vi "Verify Digraph for Simulation Mappings.vi"() -> (3 "test passed":bool)   [LabVIEW 2015]
uses:
  GraphViz Mapping Visualizer.lvlib
  <vilib>/NI/Tag Bus/tag/Data Type.ctl
  <vilib>/NI/Tag Bus/tag/tag descriptor.lvclass
panel:
  out "digraph output":string
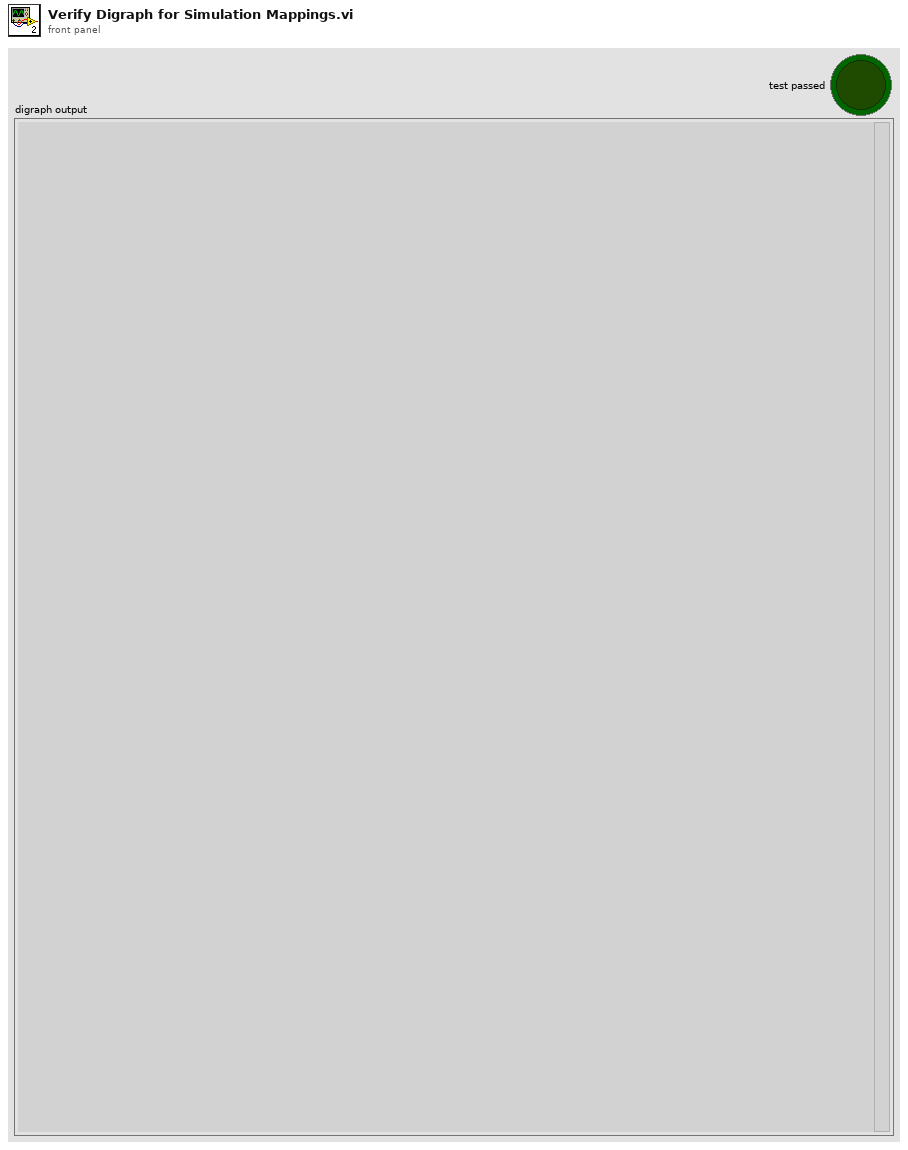
[diagram p1: front panel]
types:
  T1 = cluster{"Instance ID":string, "name":string, "default value string":string, "index":i32}[]
  T2 = typedef "tag bus.lvlib/tag descriptor.lvclass/Data Type.ctl" = enum16{"Double", "Single", "I64", "I32", "I16", "I8", "U64", "U32", "U16", "U8", "Boolean", "String", "Array of Double", "Array of Single", "Array of I64", "Array of I32", "Array of I16", "Array of I8", "Array of U64", "Array of U32", "Array of U16", "Array of U8", "Array of Boolean", "Array of String"}
  T3 = cluster{"name":string, "data type":T2, "writer":string, "readers":string[]}[]
  T4 = cluster{"display strings and indices":cluster{"Instance ID":string, "name":string, "default value string":string, "index":i32}[], "display strings and indices":cluster{"Instance ID":string, "name":string, "default value string":string, "index":i32}[]}
  T5 = typedef "GraphViz Mapping Visualizer.lvlib/Channel to Port Pair.ctl" = cluster{"Channel Name":string, "Node:Port":string}
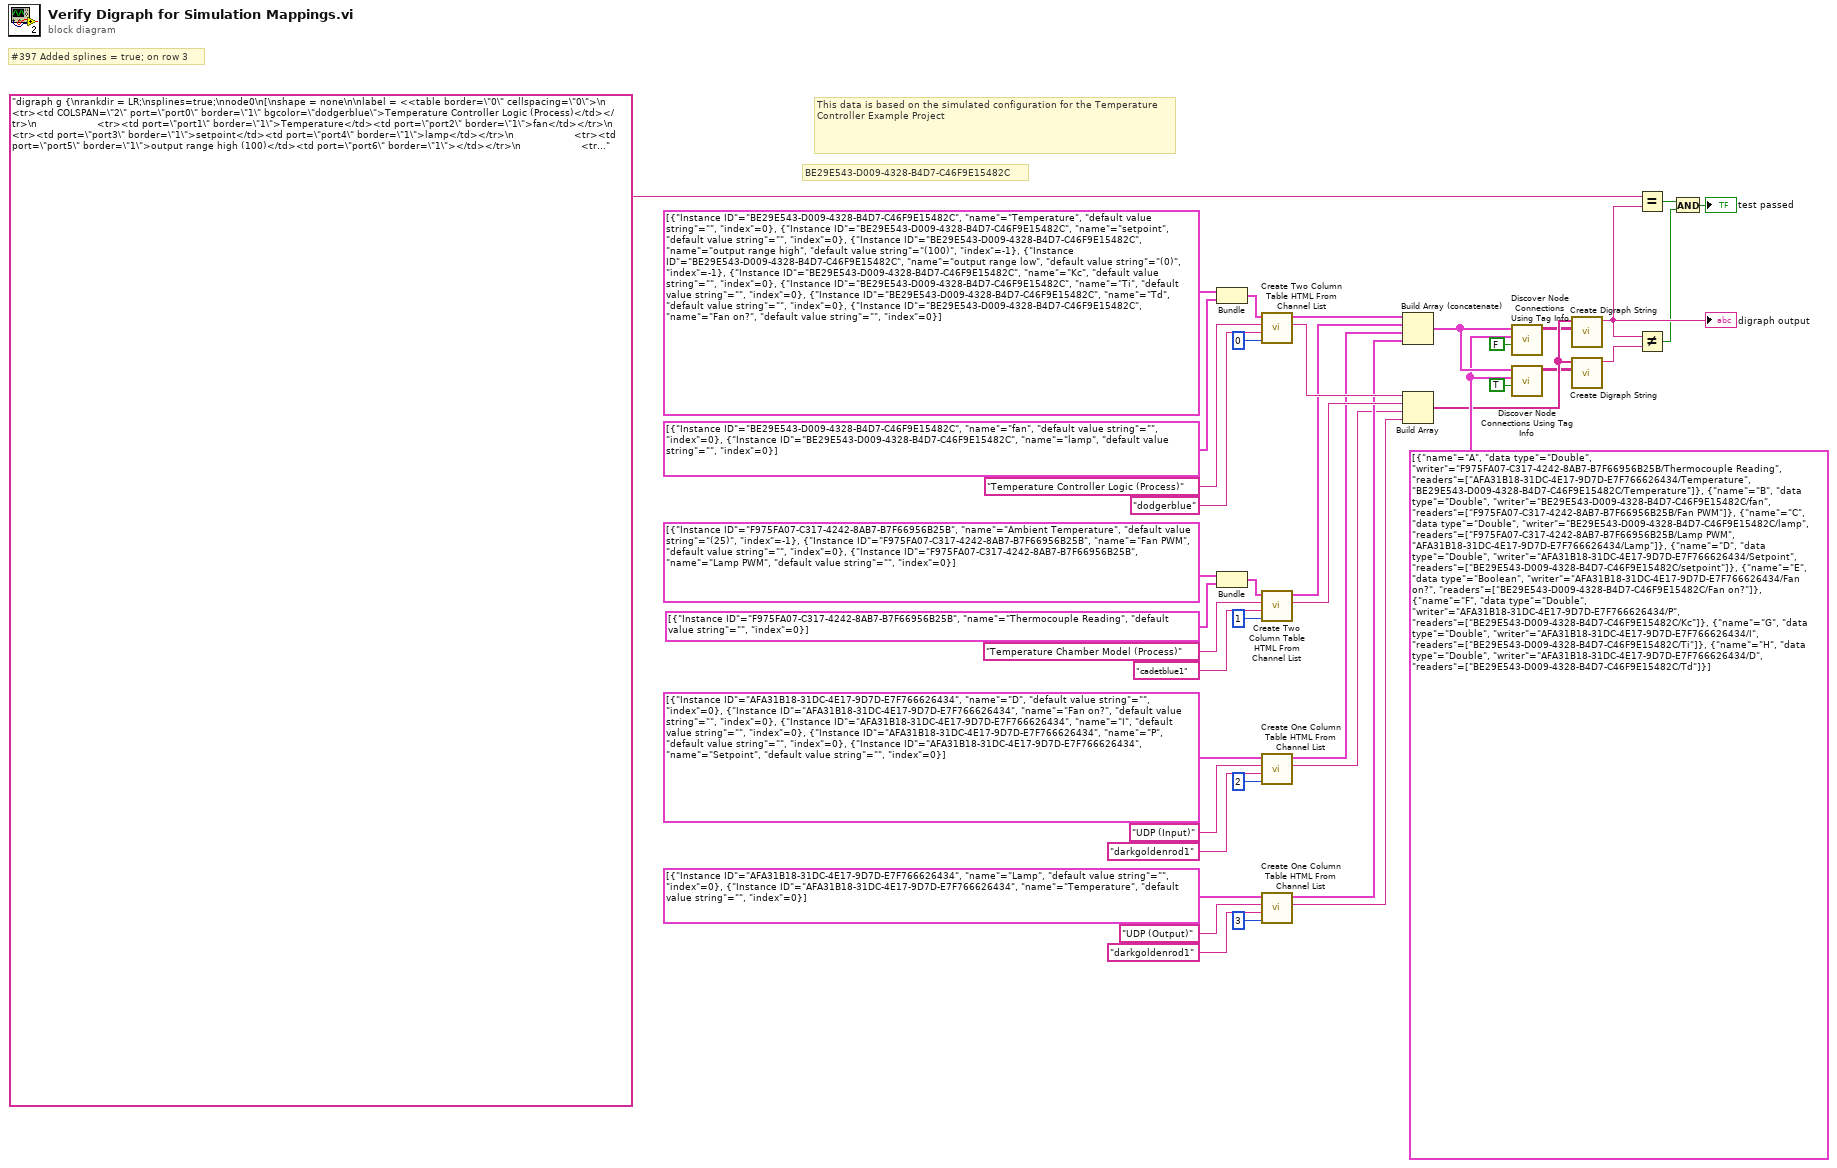
[diagram p0: block diagram]
diagram:
  w6 = T3 [{"name"="A", "data type"=enum."Double", "writer"="F975FA07-C317-4242-8AB7-B7F66956B25B/Thermocouple Reading", "readers"=["AFA31B18-31DC-4E17-9D7D-E7F766626434/Temperature", "BE29E543-D009-4328-B4D7-C46F9E15482C/Temperature"]}, {"name"="B", "data type"=enum."Double", "writer"="BE29E543-D009-4328-B4D7-C46F9E15482C/fan", "readers"=["F975FA07-C317-4242-8AB7-B7F66956B25B/Fan PWM"]}, {"name"="C", "data type"=enum."Double", "writer"="BE29E543-D009-4328-B4D7-C46F9E15482C/lamp", "readers"=["F975FA07-C317-4242-8AB7-B7F66956B25B/Lamp PWM", "AFA31B18-31DC-4E17-9D7D-E7F766626434/Lamp"]}, {"name"="D", "data type"=enum."Double", "writer"="AFA31B18-31DC-4E17-9D7D-E7F766626434/Setpoint", "readers"=["BE29E543-D009-4328-B4D7-C46F9E15482C/setpoint"]}, {"name"="E", "data type"=enum."Boolean", "writer"="AFA31B18-31DC-4E17-9D7D-E7F766626434/Fan on?", "readers"=["BE29E543-D009-4328-B4D7-C46F9E15482C/Fan on?"]}, {"name"="F", "data type"=enum."Double", "writer"="AFA31B18-31DC-4E17-9D7D-E7F766626434/P", "readers"=["BE29E543-D009-4328-B4D7-C46F9E15482C/Kc"]}, {"name"="G", "data type"=enum."Double", "writer"="AFA31B18-31DC-4E17-9D7D-E7F766626434/I", "readers"=["BE29E543-D009-4328-B4D7-C46F9E15482C/Ti"]}, {"name"="H", "data type"=enum."Double", "writer"="AFA31B18-31DC-4E17-9D7D-E7F766626434/D", "readers"=["BE29E543-D009-4328-B4D7-C46F9E15482C/Td"]}] ("tag info")
  # "#397 Added splines = true; on row 3"
  # "BE29E543-D009-4328-B4D7-C46F9E15482C"
  # "This data is based on the simulated configuration for the Temperature Controller Example Project"
  n1 = Bundle("display strings and indices"=T1 [{"Instance ID"="BE29E543-D009-4328-B4D7-C46F9E15482C", "name"="Temperature", "default value string"="", "index"=0}, {"Instance ID"="BE29E543-D009-4328-B4D7-C46F9E15482C", "name"="setpoint", "default value string"="", "index"=0}, {"Instance ID"="BE29E543-D009-4328-B4D7-C46F9E15482C", "name"="output range high", "default value string"="(100)", "index"=-1}, {"Instance ID"="BE29E543-D009-4328-B4D7-C46F9E15482C", "name"="output range low", "default value string"="(0)", "index"=-1}, {"Instance ID"="BE29E543-D009-4328-B4D7-C46F9E15482C", "name"="Kc", "default value string"="", "index"=0}, {"Instance ID"="BE29E543-D009-4328-B4D7-C46F9E15482C", "name"="Ti", "default value string"="", "index"=0}, {"Instance ID"="BE29E543-D009-4328-B4D7-C46F9E15482C", "name"="Td", "default value string"="", "index"=0}, {"Instance ID"="BE29E543-D009-4328-B4D7-C46F9E15482C", "name"="Fan on?", "default value string"="", "index"=0}], "display strings and indices"=T1 [{"Instance ID"="BE29E543-D009-4328-B4D7-C46F9E15482C", "name"="fan", "default value string"="", "index"=0}, {"Instance ID"="BE29E543-D009-4328-B4D7-C46F9E15482C", "name"="lamp", "default value string"="", "index"=0}]) -> (w20:T4)  [unwired: 1 in]
  n2 = Bundle("display strings and indices"=T1 [{"Instance ID"="F975FA07-C317-4242-8AB7-B7F66956B25B", "name"="Ambient Temperature", "default value string"="(25)", "index"=-1}, {"Instance ID"="F975FA07-C317-4242-8AB7-B7F66956B25B", "name"="Fan PWM", "default value string"="", "index"=0}, {"Instance ID"="F975FA07-C317-4242-8AB7-B7F66956B25B", "name"="Lamp PWM", "default value string"="", "index"=0}], "display strings and indices"=T1 [{"Instance ID"="F975FA07-C317-4242-8AB7-B7F66956B25B", "name"="Thermocouple Reading", "default value string"="", "index"=0}]) -> (w19:T4)  [unwired: 1 in]
  n3 = call "Create Two Column Table HTML From Channel List.vi"("Node#"=0, "Color"="dodgerblue" ("Title"), "Title"="Temperature Controller Logic (Process)", "process display strings and indices"=w20) -> ("Table HTML"=w24:string, "Channel and Node Pairs"=w25:T5[])  [unwired: 6 in]
  n4 = call "Create Two Column Table HTML From Channel List.vi"("Node#"=1, "Color"="cadetblue1" ("Title"), "Title"="Temperature Chamber Model (Process)", "process display strings and indices"=w19) -> ("Table HTML"=w12:string, "Channel and Node Pairs"=w13:T5[])  [unwired: 6 in]
  n5 = call "Create One Column Table HTML From Channel List.vi"("Node#"=2, "Color"="darkgoldenrod1" ("Title"), "Title"="UDP (Input)", "display strings and indices"=T1 [{"Instance ID"="AFA31B18-31DC-4E17-9D7D-E7F766626434", "name"="D", "default value string"="", "index"=0}, {"Instance ID"="AFA31B18-31DC-4E17-9D7D-E7F766626434", "name"="Fan on?", "default value string"="", "index"=0}, {"Instance ID"="AFA31B18-31DC-4E17-9D7D-E7F766626434", "name"="I", "default value string"="", "index"=0}, {"Instance ID"="AFA31B18-31DC-4E17-9D7D-E7F766626434", "name"="P", "default value string"="", "index"=0}, {"Instance ID"="AFA31B18-31DC-4E17-9D7D-E7F766626434", "name"="Setpoint", "default value string"="", "index"=0}]) -> ("Table HTML"=w9:string, "Channel and Node Pairs"=w11:T5[])  [unwired: 6 in]
  n6 = call "Create One Column Table HTML From Channel List.vi"("Node#"=3, "Color"="darkgoldenrod1" ("Title"), "Title"="UDP (Output)", "display strings and indices"=T1 [{"Instance ID"="AFA31B18-31DC-4E17-9D7D-E7F766626434", "name"="Lamp", "default value string"="", "index"=0}, {"Instance ID"="AFA31B18-31DC-4E17-9D7D-E7F766626434", "name"="Temperature", "default value string"="", "index"=0}]) -> ("Table HTML"=w8:string, "Channel and Node Pairs"=w10:T5[])  [unwired: 6 in]
  n7 = Build Array (concatenate)(w25, w13, w11, w10) -> (w7:T5[])
  n8 = Build Array(w24, w12, w9, w8) -> (w3:string[])
  n9 = call "Discover Node Connections Using Tag Info.vi"("Show Tag Labels?"=FALSE, "tag info"=w6, "channel and node pairs"=w7) -> ("node connections"=w2:string[][])  [unwired: 8 in]
  n10 = call "Discover Node Connections Using Tag Info.vi"("Show Tag Labels?"=TRUE, "tag info"=w6, "channel and node pairs"=w7) -> ("node connections"=w1:string[][])  [unwired: 8 in]
  n11 = call "Create Digraph String.vi"("node connections"=w2, "tables html"=w3) -> ("digraph output"=w32:string)  [unwired: 9 in]
  "digraph output" <- w32
  n12 = call "Create Digraph String.vi"("node connections"=w1, "tables html"=w3) -> ("digraph output"=w31:string)  [unwired: 9 in]
  n13 = Equal?(x="digraph g {\nrankdir = LR;\nsplines=true;\nnode0\n[\nshape = none\n\nlabel = <<table border=\"0\" cellspacing=\"0\">\n                    <tr><td COLSPAN=\"2\" port=\"port0\" border=\"1\" bgcolor=\"dodgerblue\">Temperature Controller Logic (Process)</td></tr>\n                    <tr><td port=\"port1\" border=\"1\">Temperature</td><td port=\"port2\" border=\"1\">fan</td></tr>\n                    <tr><td port=\"port3\" border=\"1\">setpoint</td><td port=\"port4\" border=\"1\">lamp</td></tr>\n                    <tr><td port=\"port5\" border=\"1\">output range high (100)</td><td port=\"port6\" border=\"1\"></td></tr>\n                    <tr><td port=\"port7\" border=\"1\">output range low (0)</td><td port=\"port8\" border=\"1\"></td></tr>\n                    <tr><td port=\"port9\" border=\"1\">Kc</td><td port=\"port10\" border=\"1\"></td></tr>\n                    <tr><td port=\"port11\" border=\"1\">Ti</td><td port=\"port12\" border=\"1\"></td></tr>\n                    <tr><td port=\"port13\" border=\"1\">Td</td><td port=\"port14\" border=\"1\"></td></tr>\n                    <tr><td port=\"port15\" border=\"1\">Fan on?</td><td port=\"port16\" border=\"1\"></td></tr>\n</table>>\n]\nnode1\n[\nshape = none\n\nlabel = <<table border=\"0\" cellspacing=\"0\">\n                    <tr><td COLSPAN=\"2\" port=\"port0\" border=\"1\" bgcolor=\"cadetblue1\">Temperature Chamber Model (Process)</td></tr>\n                    <tr><td port=\"port1\" border=\"1\">Ambient Temperature (25)</td><td port=\"port2\" border=\"1\">Thermocouple Reading</td></tr>\n                    <tr><td port=\"port3\" border=\"1\">Fan PWM</td><td port=\"port4\" border=\"1\"></td></tr>\n                    <tr><td port=\"port5\" border=\"1\">Lamp PWM</td><td port=\"port6\" border=\"1\"></td></tr>\n</table>>\n]\nnode2\n[\nshape = none\n\nlabel = <<table border=\"0\" cellspacing=\"0\">\n                    <tr><td port=\"port0\" border=\"1\" bgcolor=\"darkgoldenrod1\">UDP (Input)</td></tr>\n                    <tr><td port=\"port1\" border=\"1\">D</td></tr>\n                    <tr><td port=\"port2\" border=\"1\">Fan on?</td></tr>\n                    <tr><td port=\"port3\" border=\"1\">I</td></tr>\n                    <tr><td port=\"port4\" border=\"1\">P</td></tr>\n                    <tr><td port=\"port5\" border=\"1\">Setpoint</td></tr>\n</table>>\n]\nnode3\n[\nshape = none\n\nlabel = <<table border=\"0\" cellspacing=\"0\">\n                    <tr><td port=\"port0\" border=\"1\" bgcolor=\"darkgoldenrod1\">UDP (Output)</td></tr>\n                    <tr><td port=\"port1\" border=\"1\">Lamp</td></tr>\n                    <tr><td port=\"port2\" border=\"1\">Temperature</td></tr>\n</table>>\n]\nnode1:port2 -> node3:port2 [color=\"orange\"]\r\nnode1:port2 -> node0:port1 [color=\"orange\"]\r\nnode0:port2 -> node1:port3 [color=\"orange\"]\r\nnode0:port4 -> node1:port5 [color=\"orange\"]\r\nnode0:port4 -> node3:port1 [color=\"orange\"]\r\nnode2:port5 -> node0:port3 [color=\"orange\"]\r\nnode2:port2 -> node0:port15 [color=\"green\"]\r\nnode2:port4 -> node0:port9 [color=\"orange\"]\r\nnode2:port3 -> node0:port11 [color=\"orange\"]\r\nnode2:port1 -> node0:port13 [color=\"orange\"]\r\n}" ("String"), y=w32) -> (x = y?=w29:bool)
  n14 = Not Equal?(x=w32, y=w31) -> (x != y?=w30:bool)
  n15 = And(x=w29, y=w30) -> (x .and. y?=→"test passed":bool)
